vi "Serial_Manager_Laser.vi"(7 "Job":T1(ring), 8 "error in":errorcluster, 10 "write buffer":string, 11 "VISA resource":refnum<visa-resource-name>) -> (0 "error out":errorcluster, 2 "read buffer":string)   [LabVIEW 2011]
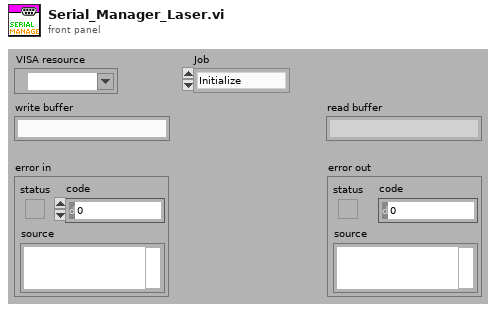
[diagram p1: front panel]
types:
  T1 = enum16{"Initialize", "Write", "Write/Read", "Read", "Clear", "Close"}
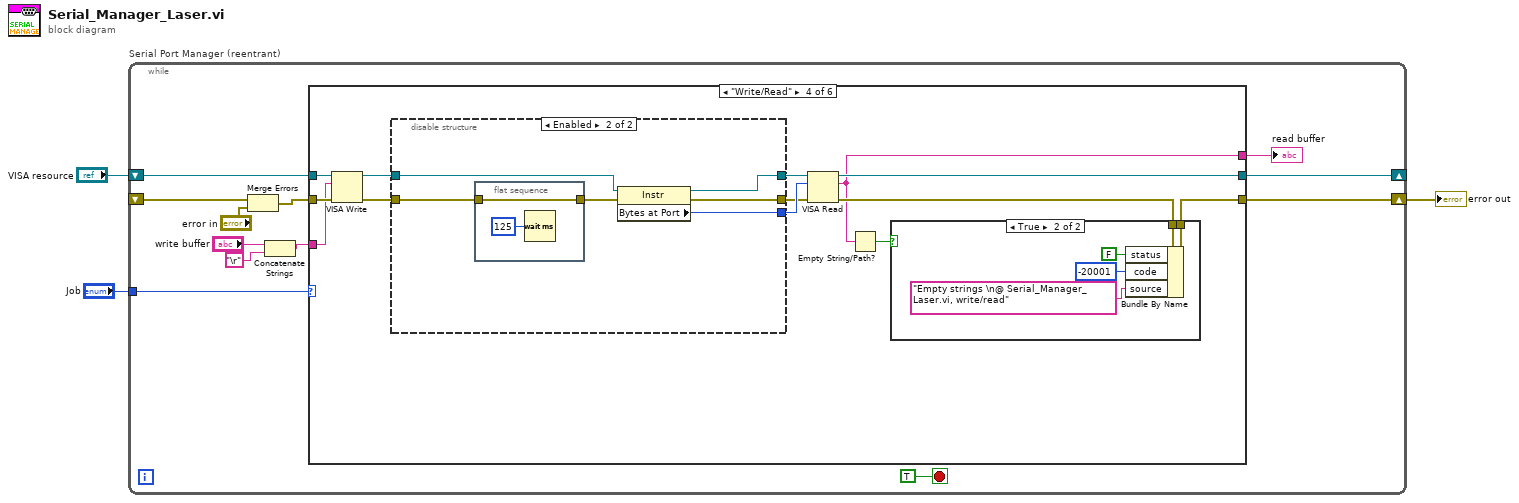
[diagram p0: block diagram]
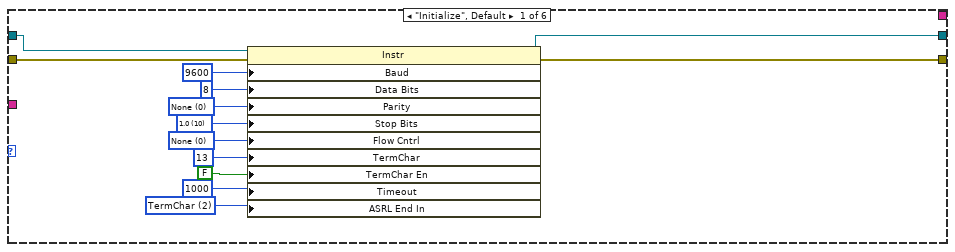
[diagram p2: hidden frame]
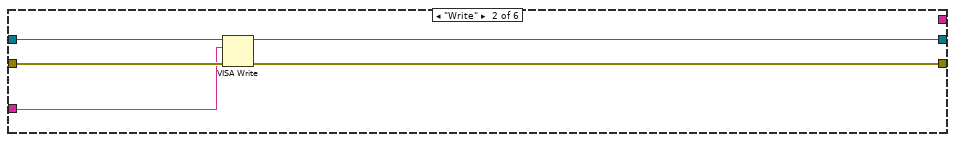
[diagram p3: hidden frame]
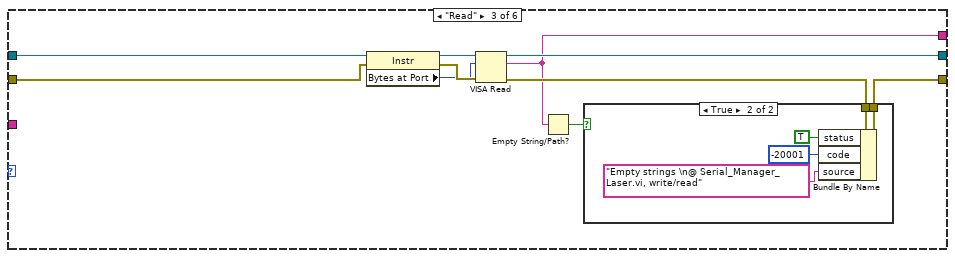
[diagram p4: hidden frame]
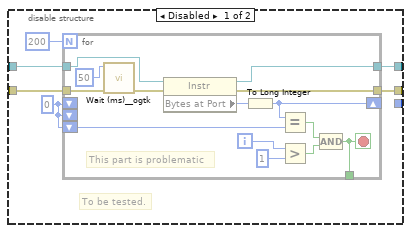
[diagram p7: hidden frame]
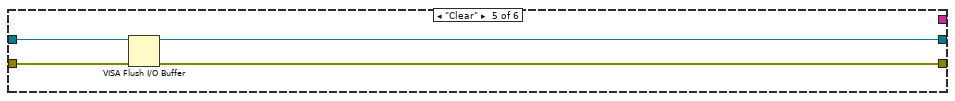
[diagram p8: hidden frame]
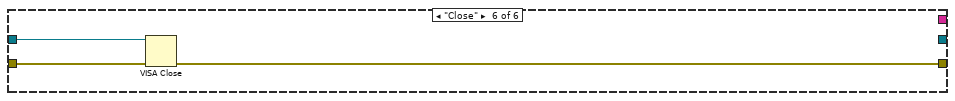
[diagram p9: hidden frame]
diagram:
  n1 = while "Serial Port Manager (reentrant)" {
    shift-right: [w14] -> _
    shift-left: "VISA resource" -> [w15]
    tunnel: "Job" -> [w13]
    shift-right: [w5] -> w1
    shift-left: _ -> [w10]
    stop <- TRUE stop-if-true
    n2 = Merge Errors(w10, "error in") -> (w11:errorcluster)
    n3 = Concatenate Strings("write buffer", "\r") -> (w7:string)
    n4 = case shown="\"Write/Read\"" w13 {
      tunnel: w15 -> [w19 w33 w42 w60 w99 w103]
      tunnel: [w27 w30 w43 w62 w98 _] -> w14
      tunnel: [w28 w31 w36 w51 w97 w102] -> w5
      tunnel: w11 -> [w18 w32 w40 w59 w100 w101]
      tunnel: w7 -> [_ w29 _ w56 _ _]
      tunnel: [_ _ w34 w50 _ _] -> w4
      frame "Initialize", Default {
        w17 = u16 2 items=["None", "Last Bit", "TermChar"] ("Serial Settings:End Mode for Reads")
        w22 = u16 0 items=["None", "XON/XOFF", "RTS/CTS", "XON/XOFF & RTS/CTS", "DTR/DSR", "XON/XOFF & DTR/DSR"] ("Serial Settings:Flow Control")
        w23 = u16 10 items=["1.0"=10, "1.5"=15, "2.0"=20] ("Serial Settings:Stop Bits")
        w24 = u16 0 items=["None", "Odd", "Even", "Mark", "Space"] ("Serial Settings:Parity")
        n5 = property class="Instr"(reference=w19, error in=w18, "Baud"=u32 9600 ("Serial Settings:Baud Rate"), "Data Bits"=u16 8 ("Serial Settings:Data Bits"), "Parity"=w24, "Stop Bits"=w23, "Flow Cntrl"=w22, "TermChar"=u8 13 ("Message Based Settings:Termination Character"), "TermChar En"=FALSE ("Message Based Settings:Termination Character Enable"), "Timeout"=u32 1000 ("VISA Open timeout (0)"), "ASRL End In"=w17) -> (reference out=w27:refnum<visa-resource-name>, error out=w28:errorcluster)
      }
      frame "Write" {
        n6 = VISA Write(VISA resource name=w33, write buffer=w29, error in (no error)=w32) -> (VISA resource name out=w30:refnum<visa-resource-name>, error out=w31:errorcluster)  [unwired: 1 out]
      }
      frame "Read" {
        n7 = property class="Instr"(reference=w42, error in=w40) -> (reference out=w41:refnum<visa-resource-name>, error out=w39:errorcluster, "Bytes at Port"=w38:u32)
        n8 = VISA Read(VISA resource name=w41, byte count=w38, error in (no error)=w39) -> (VISA resource name out=w43:refnum<visa-resource-name>, read buffer=w34:string, error out=w35:errorcluster)  [unwired: 1 out]
        n9 = Empty String/Path?(string/path=w34) -> (empty?=w37:bool)
        n10 = case shown="True" w37 {
          tunnel: w35 -> [w44 w49]
          tunnel: [w44 w48] -> w36
          frame False {
          }
          frame True {
            n11 = Bundle By Name(cluster=w49, "status"=TRUE, "code"=-20001, "source"="Empty strings \n@ Serial_Manager_Laser.vi, write/read") -> (w48:errorcluster)
          }
        }
      }
      frame "Write/Read" {
        n12 = VISA Write(VISA resource name=w60, write buffer=w56, error in (no error)=w59) -> (VISA resource name out=w58:refnum<visa-resource-name>, error out=w57:errorcluster)  [unwired: 1 out]
        n13 = disable-structure shown="Enabled" {
          disable-tunnel: [w74 w93] -> w61
          disable-tunnel: [w73 w94] -> w54
          disable-tunnel: w58 -> [w72 w92]
          disable-tunnel: w57 -> [w71 w91]
          disable-tunnel: [_ w89] -> w55
          frame Disabled {
            w69 = 0 ("Bytes at Port")
            # "To be tested."
            n14 = for {
              N: 200 -> [_]
              tunnel: [w88] -> w74
              tunnel: [w87] -> w73
              tunnel: w72 -> [w86]
              tunnel: w71 -> [w85]
              shift-right: [w81] -> _
              shift-left: w69 -> [_]
              tunnel: [w76] -> _
              shift-left: w69 -> [_]
              shift-left: w69 -> [w75]
              i -> [w78]
              stop <- w76 stop-if-true
              # "This part is problematic"
              n15 = call <userlib>:"Wait (ms)__ogtk.vi"("error in (no error)"=w85, "milliseconds to wait"=u32 50) -> ("error out"=w84:errorcluster)  [unwired: 8 in, 1 out]
              n16 = property class="Instr"(reference=w86, error in=w84) -> (reference out=w88:refnum<visa-resource-name>, error out=w87:errorcluster, "Bytes at Port"=w82:u32)
              n17 = To Long Integer(number=w82) -> (32bit integer=w81:i32)
              n18 = Equal?(x=w81, y=w75) -> (x = y?=w80:bool)
              n19 = Greater?(x=w78, y=1) -> (0:w79:bool)
              n20 = Compound Arithmetic op=AND(w80, w79) -> (w76:bool)
            }
          }
          frame Enabled {
            n21 = flat-sequence {
              tunnel: w91 -> [w96]
              tunnel: [w96] -> w90
              frame #0 {
                n22 = Wait (ms)(milliseconds to wait=u32 125) -> ()  [unwired: 1 out]
              }
            }
            n23 = property class="Instr"(reference=w92, error in=w90) -> (reference out=w93:refnum<visa-resource-name>, error out=w94:errorcluster, "Bytes at Port"=w89:u32)
          }
        }
        n24 = VISA Read(VISA resource name=w61, byte count=w55, error in (no error)=w54) -> (VISA resource name out=w62:refnum<visa-resource-name>, read buffer=w50:string, error out=w52:errorcluster)  [unwired: 1 out]
        n25 = Empty String/Path?(string/path=w50) -> (empty?=w53:bool)
        n26 = case shown="True" w53 {
          tunnel: w52 -> [w63 w68]
          tunnel: [w63 w67] -> w51
          frame False {
          }
          frame True {
            n27 = Bundle By Name(cluster=w68, "status"=FALSE, "code"=-20001, "source"="Empty strings \n@ Serial_Manager_Laser.vi, write/read") -> (w67:errorcluster)
          }
        }
      }
      frame "Clear" {
        n28 = VISA Flush I/O Buffer(VISA resource name=w99, error in (no error)=w100) -> (VISA resource name out=w98:refnum<visa-resource-name>, error out=w97:errorcluster)  [unwired: 1 in]
      }
      frame "Close" {
        n29 = VISA Close(VISA resource name=w103, error in (no error)=w101) -> (error out=w102:errorcluster)
      }
    }
    "read buffer" <- w4
  }
  "error out" <- w1
